vi "Load New Bitfile.vi"(7 "Group":bool, 8 "error in (no error)":errorcluster, 10 "NewVal":path, 11 "Item Ref in":T1 format="%.0x") -> (0 "error out":errorcluster, 3 "Section Ref out":T1 format="%.0x")   [LabVIEW 2019, in "FPGA Addon System Explorer.lvlib"]
uses:
  FPGA Addon System Explorer.lvlib
  <vilib>/NI VeriStand/Custom Device API/Custom Device Item Ref.ctl
  Addon Shared/Types/FG Action.ctl
  Addon Shared/SubVIs/Constants.vi
  <vilib>/NI VeriStand/Custom Device Tools/Custom Device Utility Library/NI VeriStand - Search for Item by GUID.vi
  <vilib>/NI/NI VeriStand Advanced SysDef API/SysDef API/SysDef.Property.Get.vi
  <vilib>/NI/NI VeriStand Advanced SysDef API/_SubVIs/SysDef.Property.Get.Variant.vi
  <vilib>/NI/NI VeriStand Advanced SysDef API/SysDef API/SysDef.Property.Set.vi
  <vilib>/NI/NI VeriStand Advanced SysDef API/_SubVIs/SysDef.Property.Set.Variant.vi
  <vilib>/NI VeriStand/Custom Device Tools/Custom Device Utility Library/Custom Device Utility Library.lvlib
  Addon Shared/FPGA Addon Shared.lvlib
  <vilib>/NI VeriStand/Custom Device API/Custom Device API.lvlib
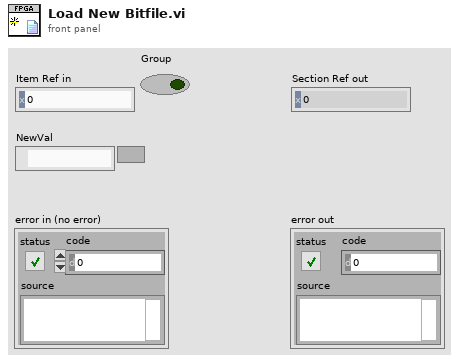
[diagram p1: front panel]
types:
  T1 = typedef "Custom Device API.lvlib/Custom Device Item Ref.ctl" = u64
  T2 = typedef "FPGA Addon Shared.lvlib/FG Action.ctl" = enum8{"GET", "SET"}
  T3 = typedef "Fifo_DMA_Config.ctl" = cluster{"Name":string, "Depth":u32, "Write? (Deprecated:Use Implementation)":bool, "Physical Channel":u32, "Base Address":u32, "Data Width":u32, "Data Type":T4, "FXP Properties":variant, "Write Window Address":u32, "Implementation":T5, "Control Set":u32}
  T4 = typedef "niFpgaDataTypeControl.ctl" = enum32{"Boolean", "I8", "I16", "I32", "I64", "U8", "U16", "U32", "U64", "FXP", "CustomControl", "SGL"}
  T5 = typedef "niFpgaDmaChannelImplementation.ctl" = enum16{"niFpgaTargetToHost", "niFpgaHostToTarget", "niFpgaPeerToPeerWriter", "niFpgaPeerToPeerReader", "niCoreTargetToHost", "niCoreHostToTarget"}
  T6 = typedef "niFpgaBitfileStructure_VI.ctl" = cluster{"Name":string, "RegisterMap":T7[], "Icon":T12}
  T7 = typedef "nirviControlStructure.ctl" = cluster{"Name":string, "Hidden":bool, "Indicator":bool, "Flattened Type":string, "Grouping":cluster{"Grouped":bool, "Member Names":string[], "Member IDs":u32[]}, "Address":u32, "Size":u32, "Class":u32, "Internal":bool, "Typedef":T8, "ID":u32, "Bidirectional":bool, "Synchronous":bool, "Mechanical Action":T9, "Sub Controls":T10[], "Access May Timeout":bool, "Register Node":bool}
  T8 = typedef "nirviTypdefDescription.ctl" = cluster{"Typedef":bool, "Path":path}
  T9 = typedef "nirviMechanicalAction.ctl" = enum8{"Switch When Pressed", "Switch When Released", "Switch Until Released", "Latch When Pressed", "Latch When Released", "Latch Until Released"}
  T10 = typedef "nirviSubControlStructure.ctl" = cluster{"Name":string, "flattened Type":string, "Cluster Information":T11, "Typedef":T8}
  T11 = typedef "nirviClusterElementControl.ctl" = cluster{"Name Hierarchy":string[], "Item Order":u32[]}
  T12 = typedef "imagedata.ctl" = cluster{"image type":i32, "image depth":i32, "image":u8[], "mask":u8[], "colors":u32[], "Rectangle":cluster{"left":i16, "top":i16, "right":i16, "bottom":i16}}
  T13 = typedef "FPGA Addon Shared.lvlib/Register Information.ctl" = cluster{"Name":string, "Data Type":T14, "Default Value":variant}
  T14 = typedef "FPGA Addon Shared.lvlib/Data Type.ctl" = enum8{"<Null>", "I8", "I16", "I32", "I64", "U8", "U16", "U32", "U64", "SGL", "Boolean", "Analog PWM In Settings", "Analog PWM In", "Digital PWM In Settings", "Digital PWM In", "Digital PWM Out", "Sine Out", "FXP+/-24.5", "FXP+/-16.5", "FXP+/-32.8", "FXP+/-64.32", "FXP+/-16.7", "FXP+/-20.5", "FXP+/-27.5", "FXP+/-32.16", "FXP+16.3", "FXP+18.3", "Digital Static In", "Digital Static Out", "Digital Static In Settings", "Digital WSS Out", "Quad Encoder Settings", "Quad Encoder In", "Group"}
  T15 = typedef "FPGA Addon Shared.lvlib/DMA Information.ctl" = cluster{"Name":string, "Data Type":T14}
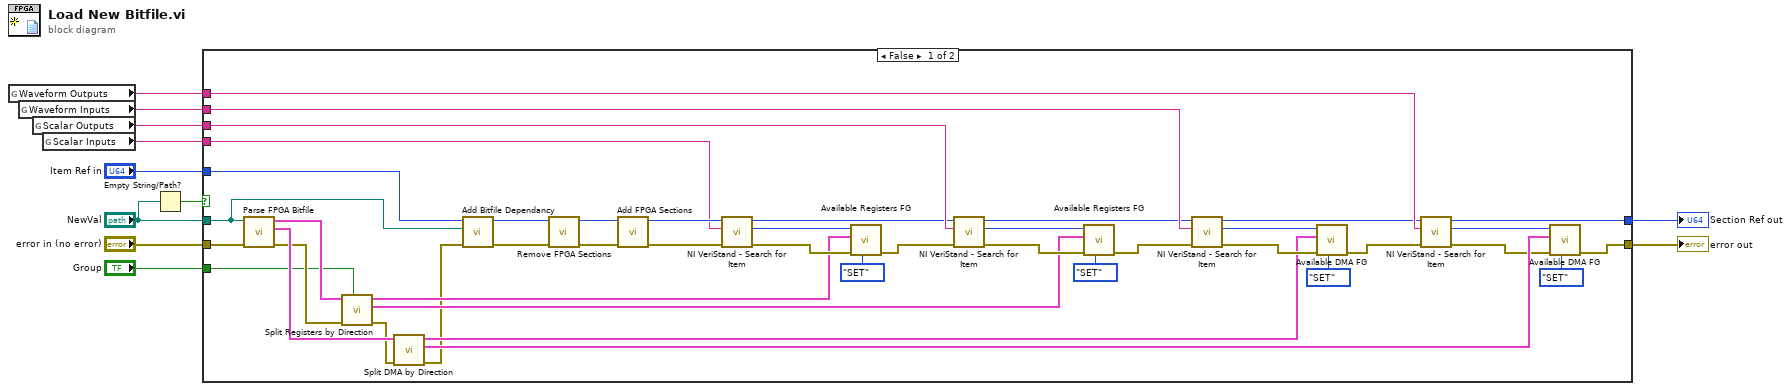
[diagram p0: block diagram]
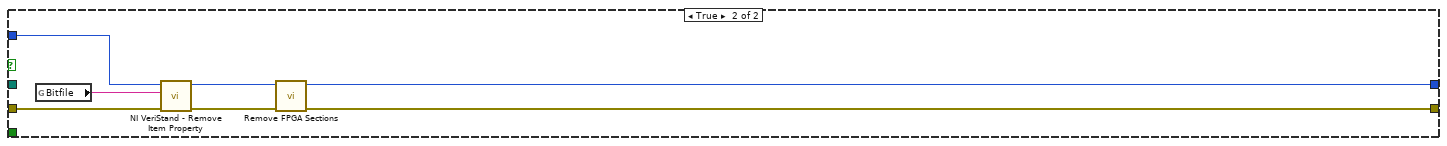
[diagram p2: hidden frame]
diagram:
  n1 = global read "Constants.vi" "Waveform Outputs"() -> (w8:string)
  n2 = global read "Constants.vi" "Waveform Inputs"() -> (w9:string)
  n3 = global read "Constants.vi" "Scalar Outputs"() -> (w10:string)
  n4 = global read "Constants.vi" "Scalar Inputs"() -> (w11:string)
  n5 = Empty String/Path?(string/path="NewVal") -> (empty?=w5:bool)
  n6 = case shown="False" w5 {
    tunnel: "NewVal" -> [w20 _]
    tunnel: "error in (no error)" -> [w54 w56]
    tunnel: w11 -> [w49 _]
    tunnel: w10 -> [w46 _]
    tunnel: w9 -> [w42 _]
    tunnel: w8 -> [w41 _]
    tunnel: [w26 w61] -> w7
    tunnel: [w24 w60] -> w6
    tunnel: "Item Ref in" -> [w19 w58]
    tunnel: "Group" -> [w12 _]
    frame False {
      n7 = call "Parse FPGA Bitfile.vi"("error in (no error)"=w54, "Path"=w20) -> ("error out"=w15:errorcluster, "DMA configuration array"=w48:T3[], "vi info"=w47:T6)  [unwired: 7 in]
      n8 = call "Split Registers by Direction.vi"("Group"=w12, "error in"=w15, "vi info"=w47) -> ("error out"=w14:errorcluster, "Controls"=w16:T13[], "Indicator"=w17:T13[])  [unwired: 6 in]
      n9 = call "Split DMA by Direction.vi"("error in"=w14, "DMA configuration array"=w48) -> ("error out"=w13:errorcluster, "HostToTarget"=w28:T15[], "TargetToHost"=w33:T15[])  [unwired: 7 in]
      n10 = call "Add Bitfile Dependancy.vi"("error in (no error)"=w13, "Path"=w20, "Item Ref in"=w19) -> ("error out"=w21:errorcluster, "Item Ref out"=w18:T1)  [unwired: 7 in]
      n11 = call "Remove FPGA Sections.vi"("error in (no error)"=w21, "Item Ref in"=w18) -> ("error out"=w22:errorcluster, "Item Ref out"=w23:T1)  [unwired: 8 in]
      n12 = call "Add FPGA Sections.vi"("error in (no error)"=w22, "Node Ptr"=w23) -> ("error out"=w52:errorcluster, "Parent Ref out"=w53:T1)  [unwired: 8 in]
      n13 = call-poly <vilib>:"NI VeriStand - Search for Item.vi"("error in"=w52, "Item GUID"=w49, "Section Ref in"=w53) -> ("error out"=w51:errorcluster, "Item Ref"=w50:T1, "Section Ref out"=w44:T1)  [unwired: 5 in, 1 out]
      n14 = call "Available Registers FG.vi"("Action"=FG_Action."SET", "error in (no error)"=w51, "Available Registers"=w17, "Item Ref"=w50) -> ("error out"=w45:errorcluster)  [unwired: 5 in, 2 out]
      n15 = call-poly <vilib>:"NI VeriStand - Search for Item.vi"("error in"=w45, "Item GUID"=w46, "Section Ref in"=w44) -> ("error out"=w37:errorcluster, "Item Ref"=w36:T1, "Section Ref out"=w40:T1)  [unwired: 5 in, 1 out]
      n16 = call "Available Registers FG.vi"("Action"=FG_Action."SET", "error in (no error)"=w37, "Available Registers"=w16, "Item Ref"=w36) -> ("error out"=w35:errorcluster)  [unwired: 5 in, 2 out]
      n17 = call-poly <vilib>:"NI VeriStand - Search for Item.vi"("error in"=w35, "Item GUID"=w42, "Section Ref in"=w40) -> ("error out"=w34:errorcluster, "Item Ref"=w43:T1, "Section Ref out"=w30:T1)  [unwired: 5 in, 1 out]
      n18 = call "Available DMA FG.vi"("Action"=FG_Action."SET", "error in (no error)"=w34, "Available DMA"=w33, "Item Ref"=w43) -> ("error out"=w31:errorcluster)  [unwired: 5 in, 2 out]
      n19 = call-poly <vilib>:"NI VeriStand - Search for Item.vi"("error in"=w31, "Item GUID"=w41, "Section Ref in"=w30) -> ("error out"=w27:errorcluster, "Item Ref"=w29:T1, "Section Ref out"=w24:T1)  [unwired: 5 in, 1 out]
      n20 = call "Available DMA FG.vi"("Action"=FG_Action."SET", "error in (no error)"=w27, "Available DMA"=w28, "Item Ref"=w29) -> ("error out"=w26:errorcluster)  [unwired: 5 in, 2 out]
    }
    frame True {
      n21 = global read "Constants.vi" "Bitfile"() -> (w59:string)
      n22 = call <vilib>:"NI VeriStand - Remove Item Property.vi"("error in (no error)"=w56, "Property Name"=w59, "Item Ref in"=w58) -> ("error out"=w55:errorcluster, "Item Ref out"=w57:T1)  [unwired: 6 in, 1 out]
      n23 = call "Remove FPGA Sections.vi"("error in (no error)"=w55, "Item Ref in"=w57) -> ("error out"=w61:errorcluster, "Item Ref out"=w60:T1)  [unwired: 8 in]
    }
  }
  "error out" <- w7
  "Section Ref out" <- w6
